vi "Encoder to current.vi"(10 "Encoder velocity":dbl) -> (2 "Drive Motor current":dbl)   [LabVIEW 2017]
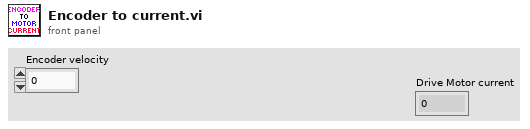
[diagram p1: front panel]
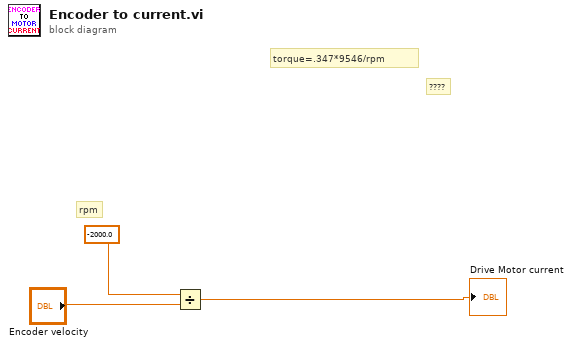
[diagram p0: block diagram]
diagram:
  # "????"
  # "rpm"
  # "torque=.347*9546/rpm"
  n1 = Divide(x=-2000.0, y="Encoder velocity") -> (x/y=→"Drive Motor current":dbl)
